vi "UpdateMotorStatus.vi"(8 "error in (MODBUS)":errorcluster, 10 "Command List":T2[](array[typedef])=[{"Reg Address"=0, "Value"=1, "Cmd/Dirrection"="START"}, {"Reg Address"=0, "Value"=0, "Cmd/Dirrection"="STOP"}, {"Reg Address"=1, "Value"=150, "Cmd/Dirrection"="TETHER IN"}, {"Reg Address"=1, "Value"=-150, "Cmd/Dirrection"="TETHER OUT"}] {"Value" min=-1000 max=1000 step=1; "Reg Address" format="%04x"}, 11 "Registers":i16[](array[numeric])=[0, 150]) -> (0 "error out (MODBUS)":errorcluster, 1 "Speed > 0?":bool, 2 "Motor State":bool, 3 "Motor Status":T1={"State"=0, "Direction"="TETHER IN", "Speed"=150} {"State" items=["OFF", "ON"]; "Speed" min=-1000 max=1000 step=1})   [LabVIEW 2018]
uses:
  Custom Controls/Address_Value Command Cluster.ctl
  Custom Controls/MotorStatusCluster.ctl
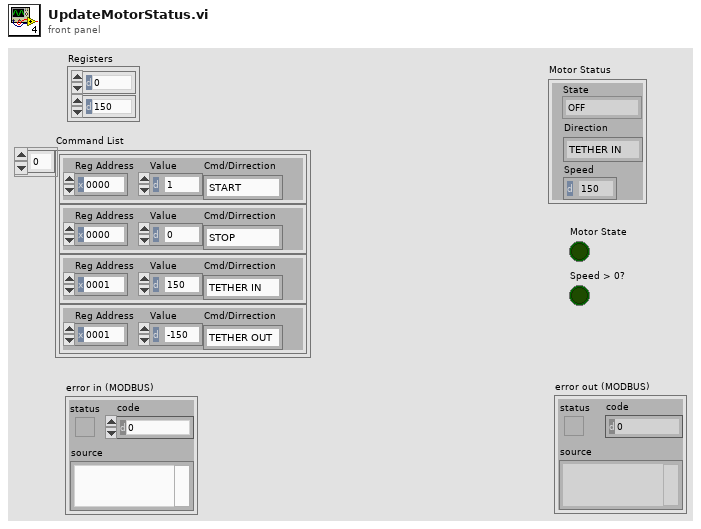
[diagram p1: front panel]
types:
  T1 = typedef "MotorStatusCluster.ctl" = cluster{"State":i16, "Direction":string, "Speed":i16}
  T2 = typedef "Address_Value Command Cluster.ctl" = cluster{"Reg Address":u16, "Value":i16, "Cmd/Dirrection":string}
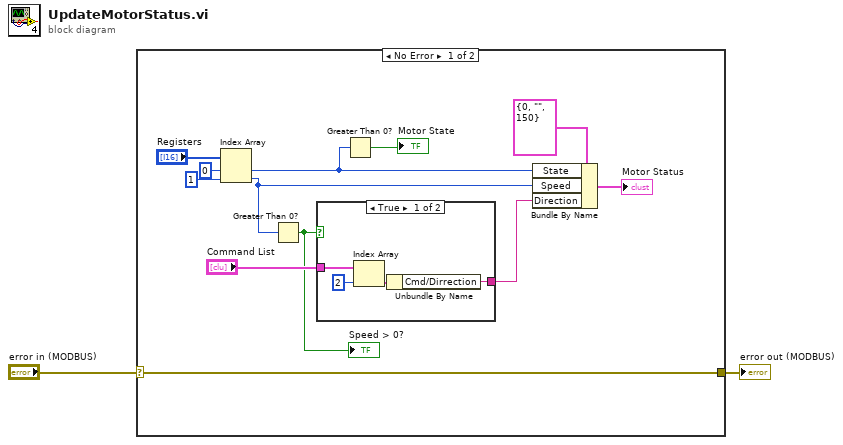
[diagram p0: block diagram]
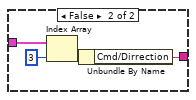
[diagram p2: hidden frame]
diagram:
  n1 = case shown="No Error" "error in (MODBUS)" {
    selector: "error in (MODBUS)" -> [w6 w23]
    tunnel: [w6 w23] -> w1
    frame No Error {
      n2 = Index Array(array="Registers", index #1=0 ("index"), index #2=1 ("index")) -> (element #1=w5:i16, element #2=w7:i16)
      n3 = Greater Than 0?(x=w7) -> (x > 0?=w3:bool)
      "Speed > 0?" <- w3
      n4 = case shown="True" w3 {
        tunnel: "Command List" -> [w18 w22]
        tunnel: [w15 w19] -> w9
        frame True {
          n5 = Index Array(array=w18, index=2) -> (element=w16:T2)
          n6 = Unbundle By Name(w16) -> ("Cmd/Dirrection"=w15:string)
        }
        frame False {
          n7 = Index Array(array=w22, index=3) -> (element=w20:T2)
          n8 = Unbundle By Name(w20) -> ("Cmd/Dirrection"=w19:string)
        }
      }
      n9 = Greater Than 0?(x=w5) -> (x > 0?=→"Motor State":bool)
      n10 = Bundle By Name(cluster=T1 {"State"=0, "Direction"="", "Speed"=150} ("Motor Status"), "State"=w5, "Speed"=w7, "Direction"=w9) -> (→"Motor Status":T1)
    }
    frame Error {
    }
  }
  "error out (MODBUS)" <- w1
